vi "Roller Step Eject.vi"() -> (0 "Close Rollers?":bool, 2 "Right Out":dbl, 3 "Left Out":dbl)   [LabVIEW 2014]
uses:
  Robot Global Data.vi
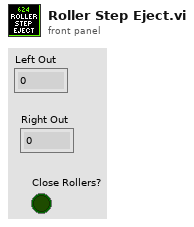
[diagram p1: front panel]
types:
  T1 = typedef "Dashboard Control Data.ctl" = cluster{"Cam Exposure":dbl, "Go to angle":dbl, "Steer PID Gains":cluster{"proportional gain (Kc)":dbl, "integral time (Ti, min)":dbl, "derivative time (Td, min)":dbl}, "Steer PID output Range":cluster{"output high":dbl, "output low":dbl}, "Pressure m \nValue":dbl, "Pressure b \nValue":dbl, "Roller Command Cluster ":T2, "Elevator":T3, "Encoder Control":T5, "Auton Settings":cluster{"Drive Dist Window Size":dbl}, "Drivetrain Settings":T6, "Lance":T7}
  T2 = typedef "Roller Control.ctl" = cluster{"Intake Speed":dbl, "Turn In Speed":dbl, "Unload Speed":dbl, "Turn Out Speed":dbl, "Ping Align Tolerance":dbl, "Tote Range Threshold":dbl, "Right Pot 0":dbl, "Pot Threshold":dbl, "Left Pot 0":dbl, "Right Pot Scale":dbl, "Left Pot Scale":dbl, "Min Elevator Height":dbl, "Eject Time":dbl, "Eject US Threshold":dbl, "Anti-Twitch Time":u32, "Ping Caring Threshold":dbl, "Pot Diff Threshold":dbl, "Pinch Sustain":u32, "Absorb Give Up Threshold":dbl, "Untip In Threshold":dbl, "Untip Grab Range":dbl, "Ultrasonic Hold Time":u32, "Landscape Absorb Time":u32, "Pot Use Wait Time":u32, "Can Turn Stop Range":dbl, "HP Load Speed":dbl, "Stick Multiplier":dbl, "Coop Eject Speed":dbl}
  T3 = typedef "Elevator DB Control.ctl" = cluster{"PID Output Range":cluster{"output high":dbl, "output low":dbl}, "PID gains":cluster{"proportional gain (Kc)":dbl, "integral time (Ti, min)":dbl, "derivative time (Td, min)":dbl}, "Height Tolerance":sgl, " Encoder Constant":dbl, "Eject Time":sgl, "Zeroing Speed":sgl, "Presets":T4, "Ping Detect Threshold":sgl, "Trashcan Detect Threshold":sgl, "Zero Filter Time":dbl, "Stabilizer Open Time":dbl, "Zero Creep Speed":dbl, "Max Current":dbl, "Current Trip Time":dbl, "Abort Pitch":dbl, "Finger m":dbl, "Finger b":dbl, "Finger max ":dbl, "Finger Stabilizer":dbl, "Finger Store":dbl, "Finger Stop Store":dbl, "Stabilizer Close Time":dbl, "Finger min":dbl, "Unstick gain":dbl, "Full Detect Max":dbl}
  T4 = typedef "Elevator Presets.ctl" = cluster{"Pickup 2 w/ Tote":sgl, "Pickup 2 w/ Trashcan":sgl, "Pickup 3 w/ Tote":sgl, "Pickup 3 w/ Trashcan":sgl, "Bottom":sgl, "Pickup 1 w/ Tote":sgl, "Pickup Trashcan":sgl, "Pickup 1 w/ Trashcan":sgl, "Eject":sgl, "Hold Low":sgl, "Step add height":sgl, "Untip Lift":dbl, "Drop Stack":dbl, "HP Load Hold":dbl, "HP Load Drop":dbl, "HP Load Hold Can":dbl, "Store can max":dbl, "HP Drag Score":dbl, "HP Drag Finish":dbl, "Finger trashcan avoid":dbl, "Full":dbl}
  T5 = typedef "Encoder Control.ctl" = cluster{"Left Tick Constant":dbl, "Right Tick Constant":dbl, "Center Tick Constant":dbl, "Reset?":bool, "Y Dist":cluster{"PID gains":cluster{"proportional gain (Kc)":dbl, "integral time (Ti, min)":dbl, "derivative time (Td, min)":dbl}}, "X Dist":cluster{"PID gains":cluster{"proportional gain (Kc)":dbl, "integral time (Ti, min)":dbl, "derivative time (Td, min)":dbl}}, "Y Stop Thresh":dbl, "Y Stop Speed":dbl, "X Stop Thresh":dbl, "X Stop Speed":dbl}
  T6 = typedef "Drivetrain Settings.ctl" = cluster{"Gyro Tolerance":sgl, "Strafe Correct max steer":sgl, "Strafe Timer Wait":sgl, "Throttle Ramp (ms)":sgl, "Strafe Ramp (ms)":sgl, "Angular rate compensation":bool, "Throttle to Rate Scale":sgl, "Rate compensation gain":sgl, "Creep Steer":sgl, "Creep Throttle":sgl}
  T7 = typedef "Pike DB Controls.ctl" = cluster{"Down Speed":dbl, "Up Speed":dbl, "Max Down Time":dbl, "Max Up Time":dbl, "Current Limit":dbl}
  T8 = typedef "Elevator Status.ctl" = cluster{"Height":dbl, "Enc Value":dbl, "Limit Override":bool, "Mode":T9, "High IR":bool, "Motor Out":dbl, "Ping Detect":bool, "Auto Elevator Indicators":T10, "Master Current":dbl, "Slave Current":dbl, "High Current":bool, "Current Tripped":bool, "Top Limit":bool, "Bottom Limit":bool, "Eject Piston":bool, "Stabilizer":bool, "Finger":bool, "Finger Height":dbl, "Finger Raw":dbl, "Finger at Bottom":bool}
  T9 = typedef "Elevator Mode.ctl" = enum16{"Manual", "Safe", "Auto"}
  T10 = typedef "Auto Elevator Indicators.ctl" = cluster{"Target Out":dbl, "Storing Trashcan?":bool, "State":T11, "In Range":bool, "Store Can Command":bool, "HP Load":bool}
  T11 = typedef "Elevator State.ctl" = enum16{"Idle", "Goto Load Position", "Wait for Load", "Load Drop", "Load Lift", "Drop Stack", "Goto Eject Position", "Eject ", "Raise Trashcan", "Open Stabilizer", "Untip Drop", "Untip Wait", "Untip Lift", "Abort Load", "HP Load Wait", "HP Load Drop", "HP Load Lift", "HP Load Abort", "Close Stabilizer", "HP Load Unfinish", "HP Load Score", "HP Load Finish", "HP Goto Finish Down", "HP Goto Finish Up", "Full"}
  T12 = typedef "Ultrasonic Indicators.ctl" = cluster{"Left Distance":dbl, "Right Distance":dbl, "Center Distance":dbl, "Left Distance Unfilter":dbl, "Right Distance Unfilter":dbl, "Center Distance Unfilter":dbl}
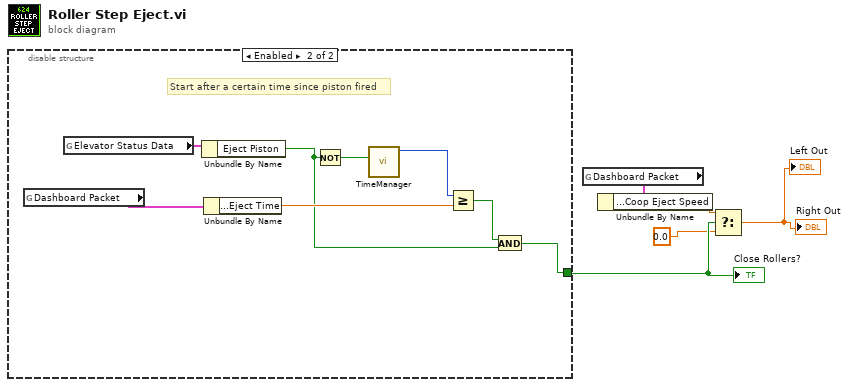
[diagram p0: block diagram]
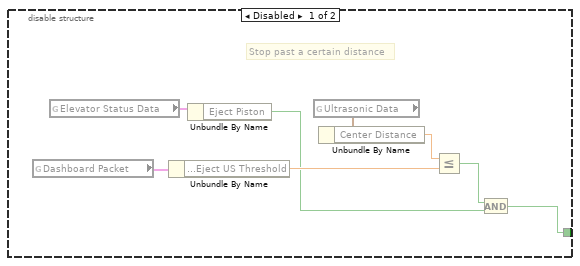
[diagram p2: hidden frame]
diagram:
  n1 = disable-structure shown="Enabled" {
    disable-tunnel: [w6 w14] -> w4
    frame Disabled {
      # "Stop past a certain distance"
      n2 = global read "Robot Global Data.vi" "Dashboard Packet"() -> (w12:T1)
      n3 = global read "Robot Global Data.vi" "Elevator Status Data"() -> (w13:T8)
      n4 = Unbundle By Name(w12) -> ("Roller Command Cluster.Eject US Threshold"=w11:dbl)
      n5 = Unbundle By Name(w13) -> ("Eject Piston"=w9:bool)
      n6 = global read "Robot Global Data.vi" "Ultrasonic Data"() -> (w8:T12)
      n7 = Unbundle By Name(w8) -> ("Center Distance"=w7:dbl)
      n8 = Less Or Equal?(x=w7, y=w11) -> (x <= y?=w10:bool)
      n9 = And(x=w10, y=w9) -> (x .and. y?=w6:bool)
    }
    frame Enabled {
      # "Start after a certain time since piston fired"
      n10 = global read "Robot Global Data.vi" "Dashboard Packet"() -> (w18:T1)
      n11 = global read "Robot Global Data.vi" "Elevator Status Data"() -> (w20:T8)
      n12 = Unbundle By Name(w20) -> ("Eject Piston"=w15:bool)
      n13 = Unbundle By Name(w18) -> ("Roller Command Cluster.Eject Time"=w17:dbl)
      n14 = Not(x=w15) -> (.not. x?=w21:bool)
      n15 = call "TimeManager.vi"("Reset?"=w21) -> ("Time Since Reset"=w19:u32)  [unwired: 9 in, 1 out]
      n16 = Greater Or Equal?(x=w19, y=w17) -> (x >= y?=w16:bool)
      n17 = And(x=w16, y=w15) -> (x .and. y?=w14:bool)
    }
  }
  "Close Rollers?" <- w4
  n18 = global read "Robot Global Data.vi" "Dashboard Packet"() -> (w5:T1)
  n19 = Unbundle By Name(w5) -> ("Roller Command Cluster.Coop Eject Speed"=w3:dbl)
  n20 = Select(t=w3, s=w4, f=0.0) -> (s? t:f=→"Left Out" →"Right Out":dbl)
